vi "Text Description.vi"(11 "LabelPrefix in":refnum<class "LabelPrefix.lvclass">) -> (2 "Description":string, 3 "LabelPrefix out":refnum<class "LabelPrefix.lvclass">)   [LabVIEW 2011, in "Messenging.lvlib" / "LabelPrefix.lvclass"]
uses:
  LabelPrefix.lvclass
  LabelPrefix.lvclass/LabelPrefix.ctl
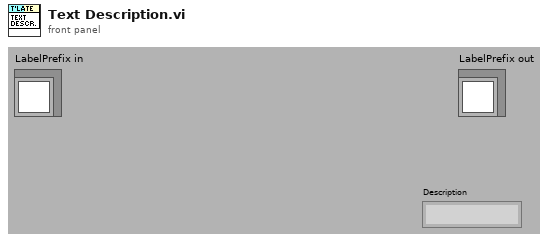
[diagram p1: front panel]
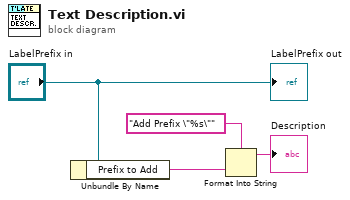
[diagram p0: block diagram]
diagram:
  n1 = Unbundle By Name("LabelPrefix in") -> ("Prefix to Add"=w2:string)
  n2 = Format Into String(format string="Add Prefix \"%s\"", w2) -> (resulting string=→"Description":string)  [unwired: 2 in, 1 out]
  "LabelPrefix out" <- "LabelPrefix in"
